vi "PeelingWB6.vi"() -> ()   [LabVIEW 2012]
uses:
  <vilib>/addons/database/Connection.llb/DB Tools Open Connec (Path).vi
  <vilib>/addons/database/Connection.llb/Conn Execute.vi
  <vilib>/addons/database/Recordset.llb/Rec Fetch Recordset Data (R).vi
  <vilib>/addons/database/Recordset.llb/Rec Destroy - Connection.vi
  <vilib>/Utility/file.llb/Write To Spreadsheet File (string).vi
  <vilib>/addons/database/_DB Variant To Data/Database Variant To Data.xnode
  <vilib>/addons/database/NI_Database_API.lvlib
panel:
  out "error out 2":errorcluster
  out "spreadsheet string":string
  out "Array 2":string[][](array[string])
  out "error out":errorcluster
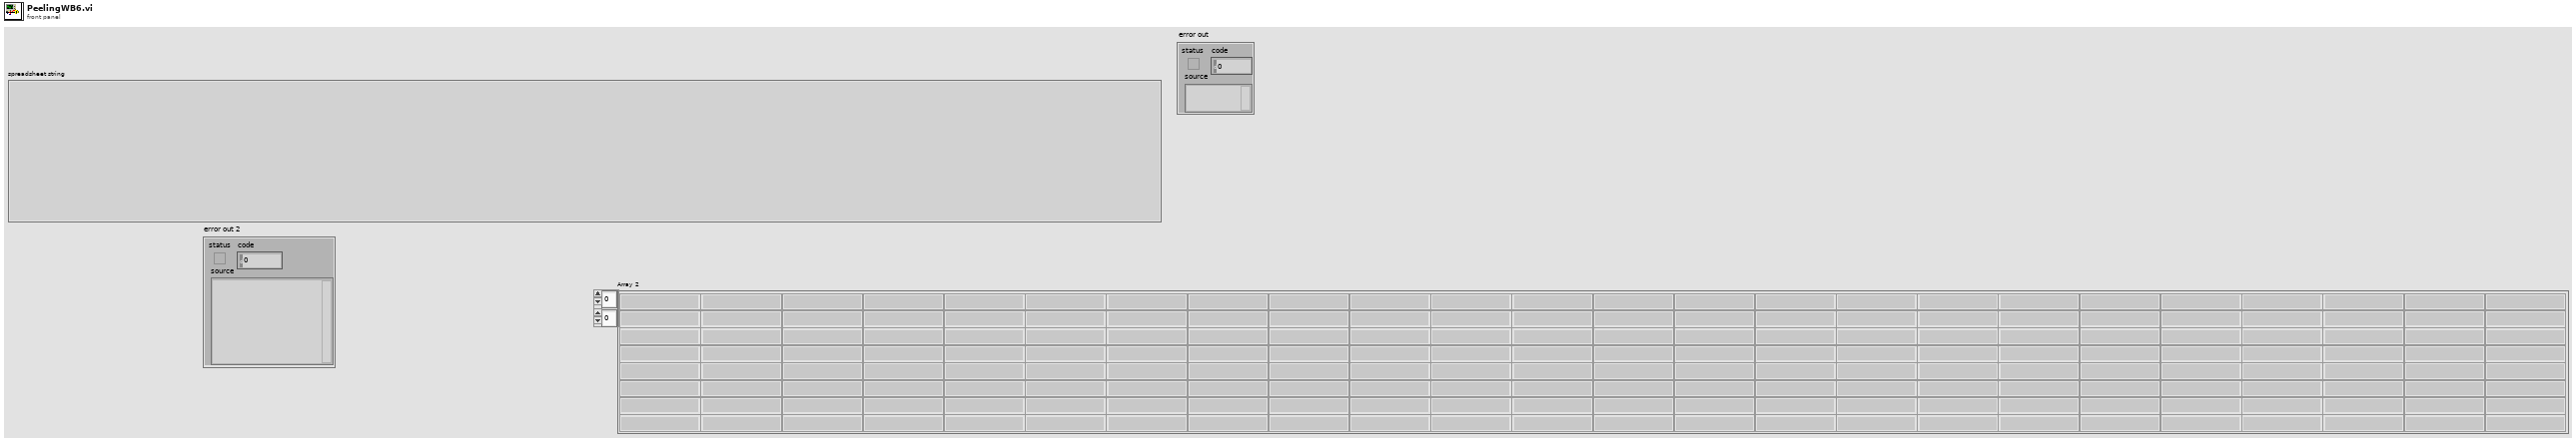
[diagram p1: front panel]
types:
  T1 = typedef "NI_Database_API.lvlib/Conn ObjectReference.ctl" = refnum<k1>
  T2 = typedef "NI_Database_API.lvlib/Rec ObjectReference.ctl" = refnum<k1>
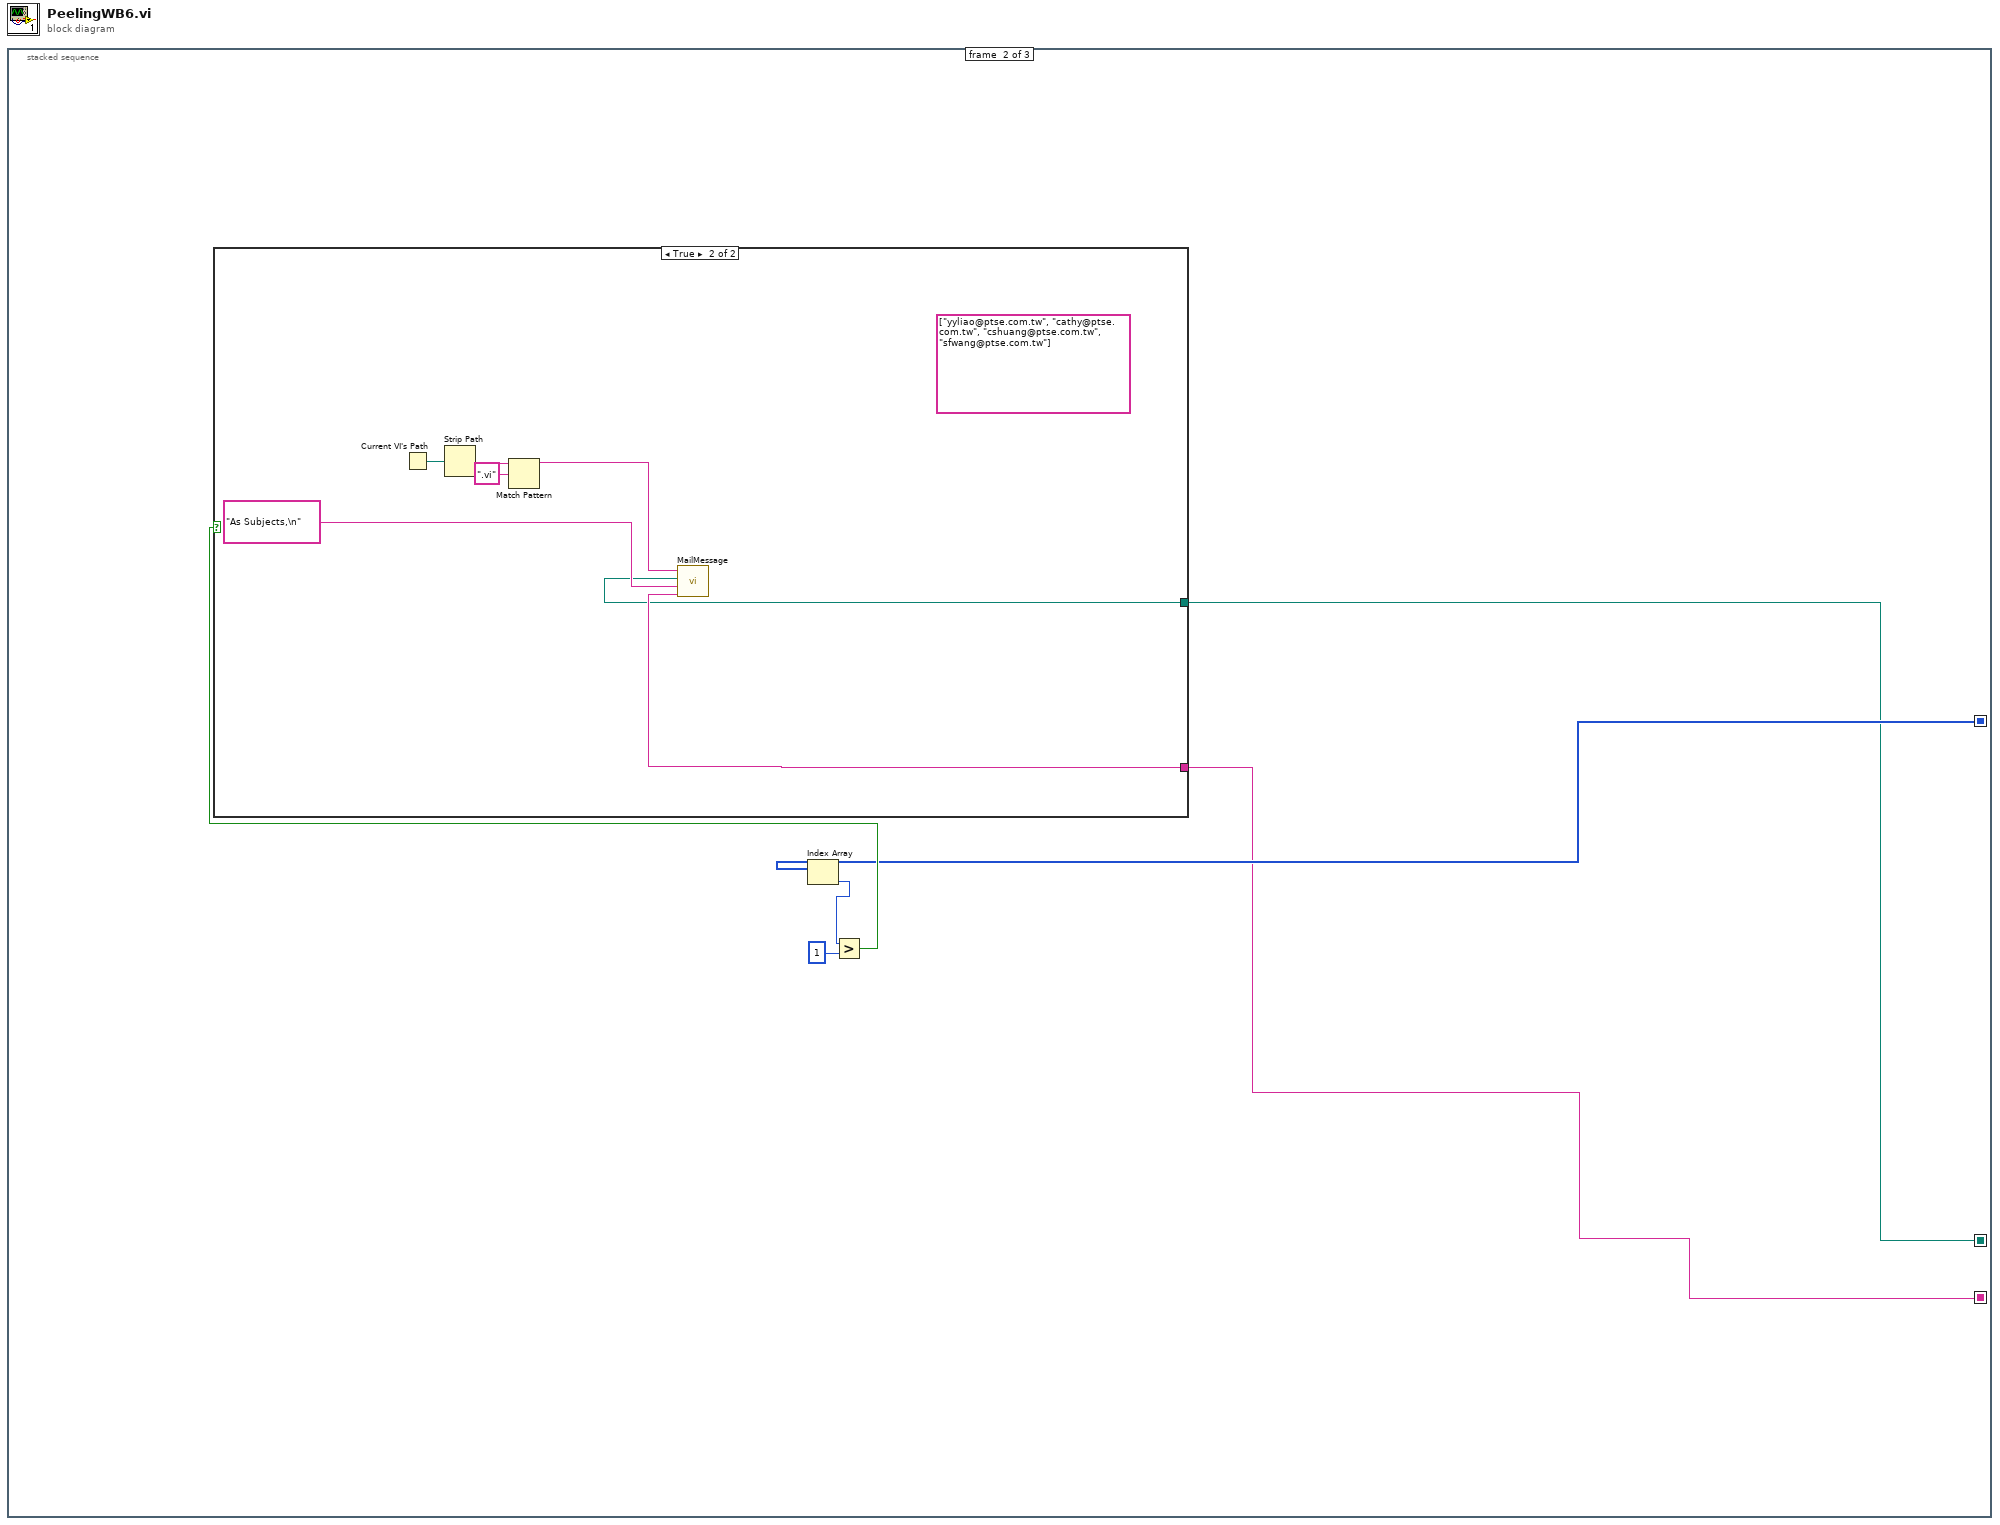
[diagram p0: block diagram]
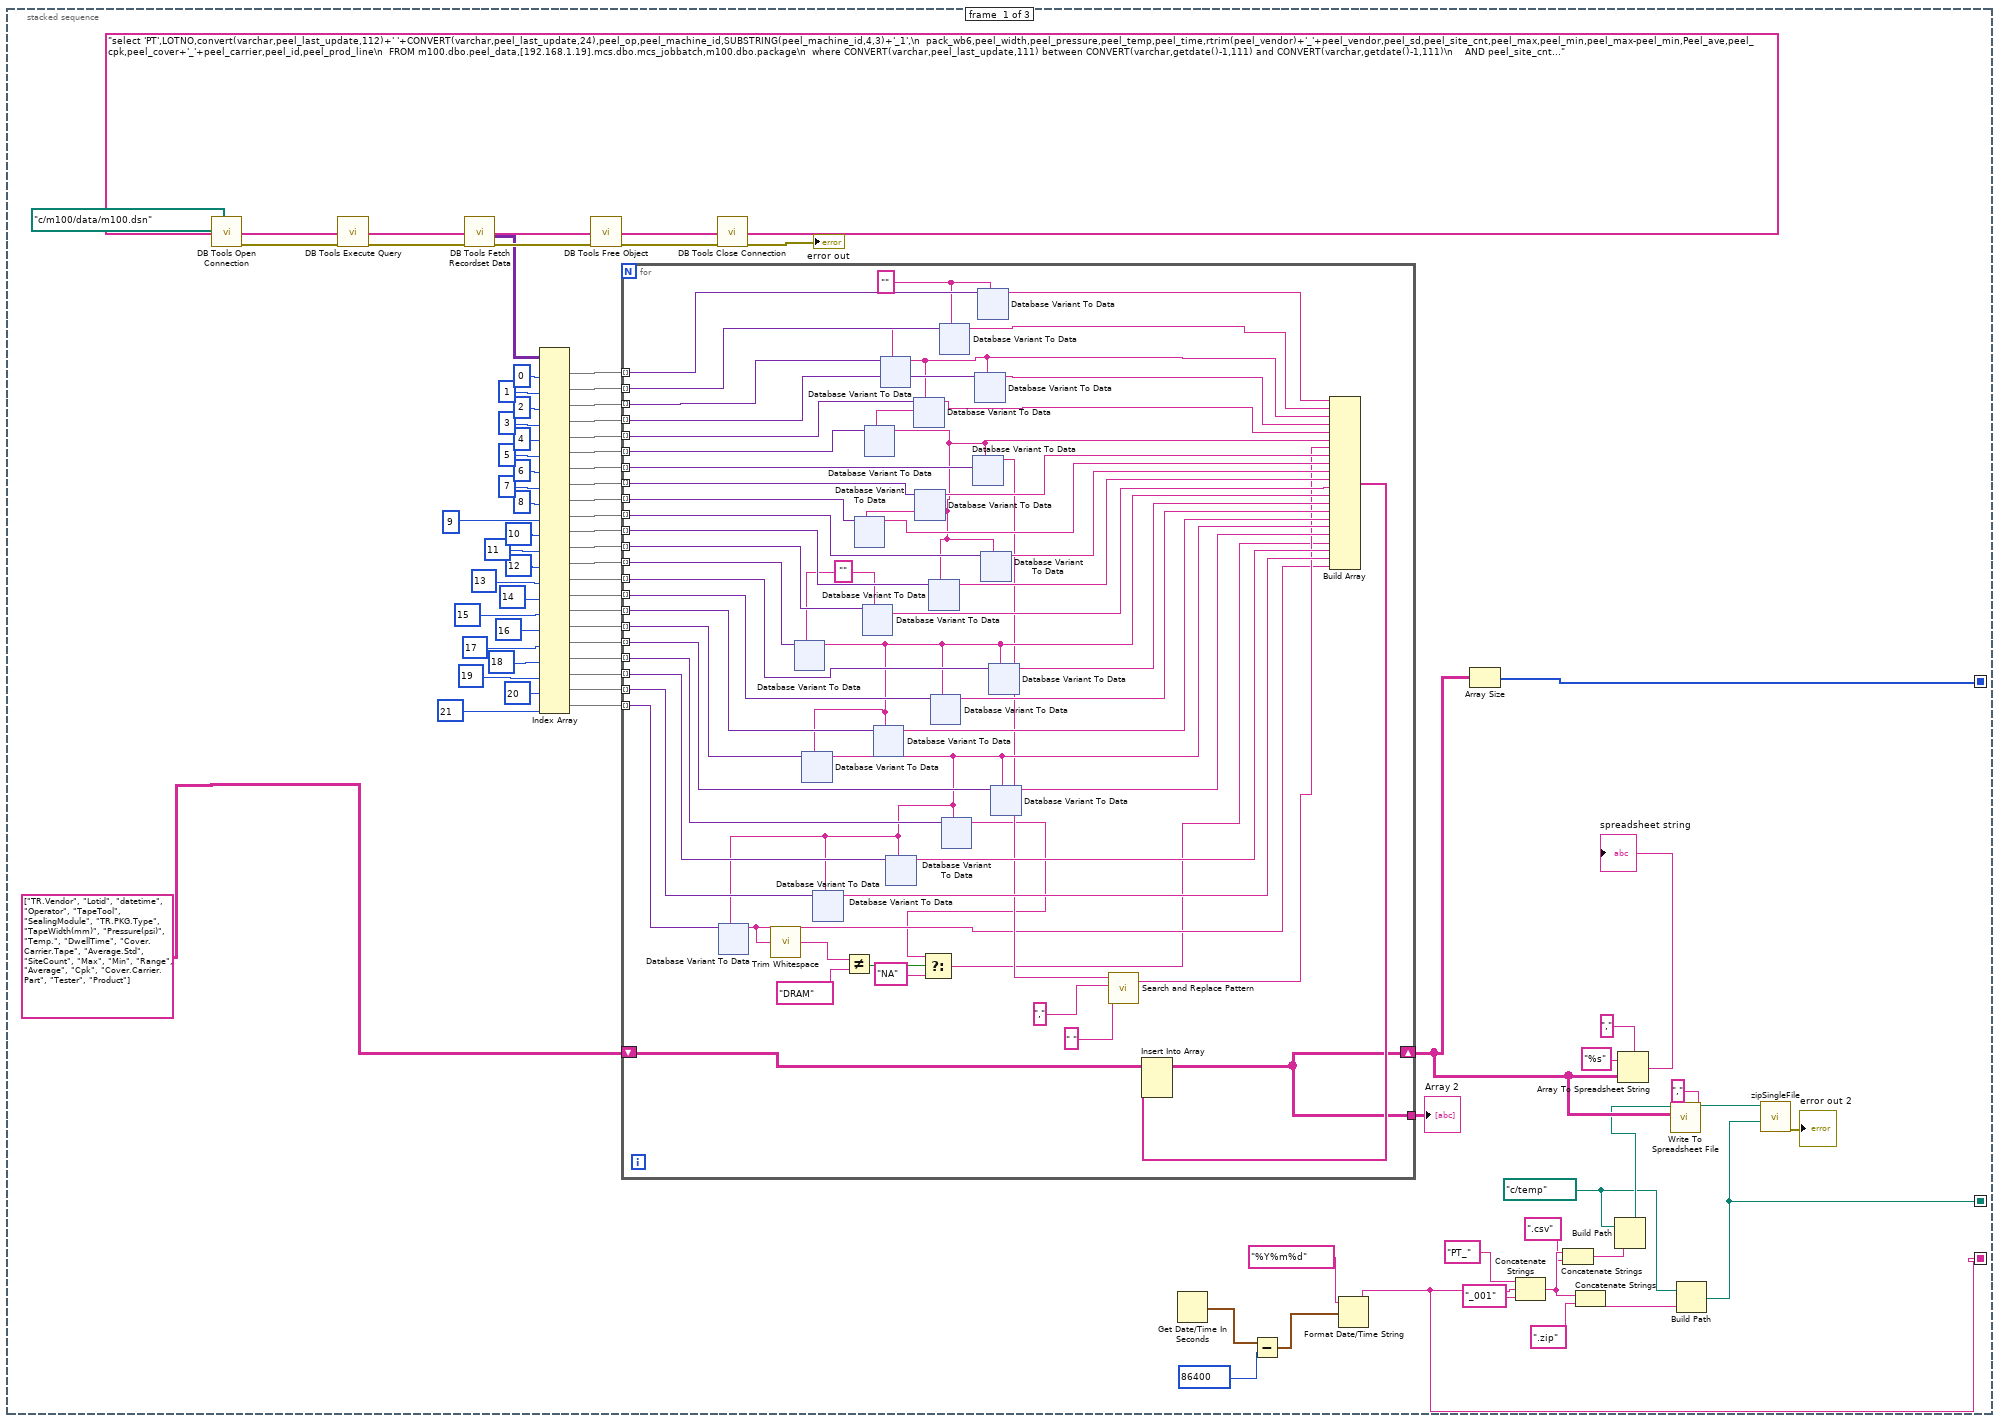
[diagram p2: hidden frame]
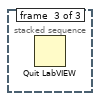
[diagram p4: hidden frame]
diagram:
  n1 = stacked-sequence {
    seq-local: [w49 _ _] -> [_ w845 _]
    seq-local: [w5 _ _] -> [_ w844 _]
    seq-local: [w4 _ _] -> [_ w843 _]
    frame #0 {
      w6 = path "c:/temp" ("base path")
      n2 = call-poly <vilib>:"DB Tools Open Connection.vi"("connection information"=path "c:/m100/data/m100.dsn") -> ("error out"=w76:errorcluster, "connection reference"=w80:T1)  [unwired: 7 in]
      n3 = call-poly <vilib>:"DB Tools Execute Query.vi"("error in (no error)"=w76, "SQL query"="select 'PT',LOTNO,convert(varchar,peel_last_update,112)+' '+CONVERT(varchar,peel_last_update,24),peel_op,peel_machine_id,SUBSTRING(peel_machine_id,4,3)+'_1',\n  pack_wb6,peel_width,peel_pressure,peel_temp,peel_time,rtrim(peel_vendor)+'_'+peel_vendor,peel_sd,peel_site_cnt,peel_max,peel_min,peel_max-peel_min,Peel_ave,peel_cpk,peel_cover+'_'+peel_carrier,peel_id,peel_prod_line\n  FROM m100.dbo.peel_data,[192.168.1.19].mcs.dbo.mcs_jobbatch,m100.dbo.package\n  where CONVERT(varchar,peel_last_update,111) between CONVERT(varchar,getdate()-1,111) and CONVERT(varchar,getdate()-1,111)\n    AND peel_site_cnt > 0\n    AND peel_result='PASS'\n    and jobno COLLATE Chinese_Taiwan_Stroke_CI_AS = peel_lot_no\n    and customerid COLLATE Chinese_Taiwan_Stroke_CI_AS='WB6'\n    and assemblytype COLLATE Chinese_Taiwan_Stroke_CI_AS = pack_pts\n    order by peel_last_update", "connection reference"=w80) -> ("error out"=w75:errorcluster, "recordset reference"=w79:T2)  [unwired: 5 in]
      n4 = call-poly <vilib>:"DB Tools Fetch Recordset Data.vi"("error in (no error)"=w75, "recordset reference"=w79) -> ("error out"=w74:errorcluster, "recordset data"=w43:variant[][], "recordset reference out"=w78:T2)  [unwired: 3 in]
      n5 = Index Array(array=w43, index (col) #1=0 ("disabled index (col)"), index (col) #2=1 ("index (col)"), index (col) #3=2 ("index (col)"), index (col) #4=3 ("index (col)"), index (col) #5=4 ("index (col)"), index (col) #6=5 ("index (col)"), index (col) #7=6 ("index (col)"), index (col) #8=7 ("index (col)"), index (col) #9=8 ("index (col)"), index (col) #10=9 ("index (col)"), index (col) #11=10 ("index (col)"), index (col) #12=11 ("index (col)"), index (col) #13=12 ("index (col)"), index (col) #14=13 ("index (col)"), index (col) #15=14 ("index (col)"), index (col) #16=15 ("index (col)"), index (col) #17=16 ("index (col)"), index (col) #18=17 ("index (col)"), index (col) #19=18 ("index (col)"), index (col) #20=19 ("index (col)"), index (col) #21=20 ("index (col)"), index (col) #22=21 ("index (col)")) -> (element #1=w60:variant[], element #2=w59:variant[], element #3=w58:variant[], element #4=w57:variant[], element #5=w56:variant[], element #6=w55:variant[], element #7=w54:variant[], element #8=w53:variant[], element #9=w52:variant[], element #10=w51:variant[], element #11=w50:variant[], element #12=w46:variant[], element #13=w45:variant[], element #14=w33:variant[], element #15=w32:variant[], element #16=w31:variant[], element #17=w30:variant[], element #18=w29:variant[], element #19=w28:variant[], element #20=w27:variant[], element #21=w26:variant[], element #22=w25:variant[])  [unwired: 22 in]
      n6 = call-poly <vilib>:"DB Tools Free Object.vi"("error in (no error)"=w74, "recordset reference"=w78) -> ("error out"=w73:errorcluster, "connection reference"=w77:T1)  [unwired: 8 in]
      n7 = for {
        tunnel: w60 -> [w138] mode=indexing
        tunnel: w59 -> [w137] mode=indexing
        tunnel: w58 -> [w136] mode=indexing
        tunnel: w57 -> [w135] mode=indexing
        tunnel: w56 -> [w134] mode=indexing
        tunnel: w55 -> [w133] mode=indexing
        tunnel: w54 -> [w132] mode=indexing
        tunnel: w53 -> [w131] mode=indexing
        tunnel: w52 -> [w130] mode=indexing
        tunnel: w51 -> [w129] mode=indexing
        tunnel: w50 -> [w128] mode=indexing
        tunnel: [w125] -> w23
        shift-right: [w125] -> w19
        shift-left: string[][] [["TR.Vendor", "Lotid", "datetime", "Operator", "TapeTool", "SealingModule", "TR.PKG.Type", "TapeWidth(mm)", "Pressure(psi)", "Temp.", "DwellTime", "Cover.Carrier.Tape", "Average.Std", "SiteCount", "Max", "Min", "Range", "Average", "Cpk", "Cover.Carrier.Part", "Tester", "Product"]] ("Array") -> [w124]
        tunnel: w46 -> [w123] mode=indexing
        tunnel: w45 -> [w122] mode=indexing
        tunnel: w33 -> [w110] mode=indexing
        tunnel: w32 -> [w109] mode=indexing
        tunnel: w31 -> [w108] mode=indexing
        tunnel: w30 -> [w107] mode=indexing
        tunnel: w29 -> [w106] mode=indexing
        tunnel: w28 -> [w105] mode=indexing
        tunnel: w27 -> [w104] mode=indexing
        tunnel: w26 -> [w103] mode=indexing
        tunnel: w25 -> [w102] mode=indexing
        w121 = ""
        w118 = ""
        n8 = xnode "Database Variant To Data"("database variant"=w122, "type"=w121) -> ("data"=w101:string)  [unwired: 1 in, 1 out]
        n9 = xnode "Database Variant To Data"("database variant"=w107, "type"=w101) -> ("data"=w96:string)  [unwired: 1 in, 1 out]
        n10 = xnode "Database Variant To Data"("database variant"=w102, "type"=w96) -> ("data"=w84:string)  [unwired: 1 in, 1 out]
        n11 = call <vilib>:"Trim Whitespace.vi"("string"=w84) -> ("trimmed string"=w85:string)  [unwired: 1 in]
        n12 = xnode "Database Variant To Data"("database variant"=w103, "type"=w96) -> ("data"=w94:string)  [unwired: 1 in, 1 out]
        n13 = Not Equal?(x=w85, y="DRAM") -> (x != y?=w87:bool)
        n14 = xnode "Database Variant To Data"("database variant"=w123, "type"=w121) -> ("data"=w120:string)  [unwired: 1 in, 1 out]
        n15 = xnode "Database Variant To Data"("database variant"=w108, "type"=w101) -> ("data"=w98:string)  [unwired: 1 in, 1 out]
        n16 = xnode "Database Variant To Data"("database variant"=w136, "type"=w118) -> ("data"=w115:string)  [unwired: 1 in, 1 out]
        n17 = xnode "Database Variant To Data"("database variant"=w133, "type"=w115) -> ("data"=w91:string)  [unwired: 1 in, 1 out]
        n18 = xnode "Database Variant To Data"("database variant"=w130, "type"=w91) -> ("data"=w113:string)  [unwired: 1 in, 1 out]
        n19 = xnode "Database Variant To Data"("database variant"=w104, "type"=w96) -> ("data"=w95:string)  [unwired: 1 in, 1 out]
        n20 = xnode "Database Variant To Data"("database variant"=w134, "type"=w115) -> ("data"=w116:string)  [unwired: 1 in, 1 out]
        n21 = xnode "Database Variant To Data"("database variant"=w131, "type"=w91) -> ("data"=w114:string)  [unwired: 1 in, 1 out]
        n22 = xnode "Database Variant To Data"("database variant"=w128, "type"=w91) -> ("data"=w111:string)  [unwired: 1 in, 1 out]
        n23 = xnode "Database Variant To Data"("database variant"=w109, "type"=w101) -> ("data"=w99:string)  [unwired: 1 in, 1 out]
        n24 = xnode "Database Variant To Data"("database variant"=w137, "type"=w118) -> ("data"=w119:string)  [unwired: 1 in, 1 out]
        n25 = xnode "Database Variant To Data"("database variant"=w105, "type"=w96) -> ("data"=w83:string)  [unwired: 1 in, 1 out]
        n26 = Select(t=w83, s=w87, f="NA") -> (s? t:f=w82:string)
        n27 = xnode "Database Variant To Data"("database variant"=w132, "type"=w91) -> ("data"=w90:string)  [unwired: 1 in, 1 out]
        n28 = xnode "Database Variant To Data"("database variant"=w135, "type"=w115) -> ("data"=w117:string)  [unwired: 1 in, 1 out]
        n29 = xnode "Database Variant To Data"("database variant"=w138, "type"=w118) -> ("data"=w127:string)  [unwired: 1 in, 1 out]
        n30 = xnode "Database Variant To Data"("database variant"=w129, "type"=w91) -> ("data"=w112:string)  [unwired: 1 in, 1 out]
        n31 = xnode "Database Variant To Data"("database variant"=w110, "type"=w101) -> ("data"=w100:string)  [unwired: 1 in, 1 out]
        n32 = xnode "Database Variant To Data"("database variant"=w106, "type"=w96) -> ("data"=w97:string)  [unwired: 1 in, 1 out]
        n33 = call <vilib>:"Search and Replace Pattern.vi"("string"=w90, "regular expression (\"\")"="," ("regular expression (\"\")"), "replace string (\"\")"=" " ("replace string (\"\")")) -> ("result string"=w89:string)  [unwired: 2 in, 1 out]
        n34 = Build Array(w127, w119, w115, w117, w116, w91, w89, w114, w113, w112, w111, w120, w101, w100, w99, w98, w96, w97, w82, w95, w94, w84) -> (w126:string[])
        n35 = Insert Into Array(array=w124, new element=w126) -> (w125:string[][])  [unwired: 2 in]
      }
      "Array 2" <- w23
      n36 = call <vilib>:"DB Tools Close Connection.vi"("error in (no error)"=w73, "connection reference"=w77) -> ("error out"=→"error out":errorcluster)  [unwired: 5 in]
      n37 = Get Date/Time In Seconds() -> (seconds since 1Jan1904=w3:timestamp)
      n38 = Subtract(x=w3, y=86400) -> (x-y=w1:timestamp)
      n39 = Format Date/Time String(time format string (%c)="%Y%m%d", seconds (now)=w1) -> (date/time string=w5:string)  [unwired: 1 in]
      n40 = Array Size(array=w19) -> (size(s)=w49:i32[])
      n41 = Concatenate Strings("PT_" ("string"), w5, "_001" ("string")) -> (w10:string)
      n42 = Concatenate Strings(w10, ".csv" ("string")) -> (w7:string)
      n43 = Concatenate Strings(w10, ".zip" ("string")) -> (w11:string)
      n44 = Build Path(base path=w6, name or relative path=w7) -> (appended path=w8:path)
      n45 = Array To Spreadsheet String(delimiter (Tab)=",", array=w19, 3:"%s" ("format string")) -> (spreadsheet string=→"spreadsheet string":string)
      n46 = call-poly <vilib>:"Write To Spreadsheet File.vi"("delimiter (\\t)"="," ("delimiter (\\t)"), "2D data"=w19, "file path (dialog if empty)"=w8) -> ("new file path (Not A Path if cancelled)"=w17:path)  [unwired: 5 in]
      n47 = Build Path(base path=w6, name or relative path=w11) -> (appended path=w4:path)
      n48 = call "zipSingleFile.vi"("zip folderFile"=w4, "source file path"=w17) -> ("error out"=→"error out 2":errorcluster)  [unwired: 9 in]
    }
    frame #1 {
      n49 = Index Array(array=w845) -> (element=w848:i32)  [unwired: 1 in]
      n50 = Greater?(x=w848, y=1) -> (0:w846:bool)
      n51 = case shown="True" w846 {
        tunnel: w843 -> [_ w850]
        tunnel: w844 -> [_ w854]
        frame False {
        }
        frame True {
          (unwired) string[] ["yyliao@ptse.com.tw", "cathy@ptse.com.tw", "cshuang@ptse.com.tw", "sfwang@ptse.com.tw"] ("recipients")
          n52 = Current VI's Path() -> (path=w853:path)
          n53 = Strip Path(path=w853) -> (name=w852:string)  [unwired: 1 out]
          n54 = Match Pattern(string=w852, regular expression=".vi") -> (before substring=w849:string)  [unwired: 1 in, 3 out]
          n55 = call "MailMessage.vi"("AddSubject"=w854, "message"="As Subjects,\n", "file path"=w850, "program"=w849) -> ()  [unwired: 8 in]
        }
      }
    }
    frame #2 {
      n56 = Quit LabVIEW() -> ()  [unwired: 1 in]
    }
  }
